vi "Close.vi"(8 "error in (no error)":errorcluster, 11 "Pound":refnum<class "Pound.lvclass">) -> (0 "error out":errorcluster)   [LabVIEW 2017, in "Pound.lvclass"]
doc: "Close reference to the pound and any watchdogs that are associated with it."
uses:
  <vilib>/NI/Software Watchdog/Pound/Pound.lvclass
  <vilib>/NI/Software Watchdog/Pound/Pound.lvclass/Pound.ctl
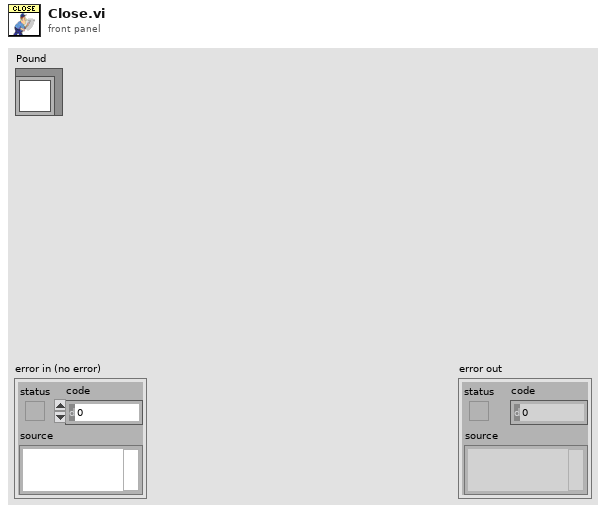
[diagram p1: front panel]
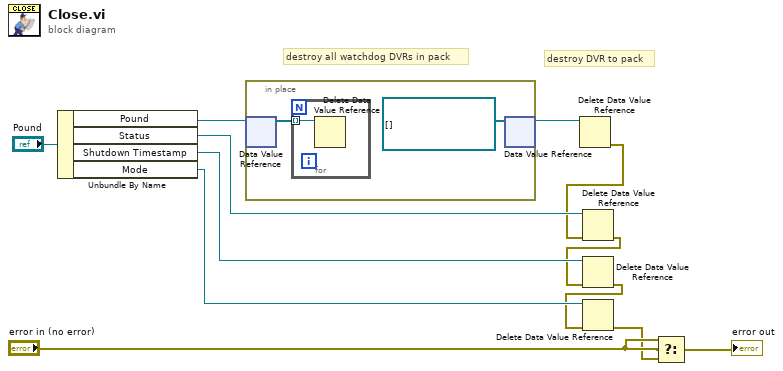
[diagram p0: block diagram]
diagram:
  # "destroy all watchdog DVRs in pack"
  # "destroy DVR to pack"
  n1 = Unbundle By Name("Pound") -> ("Pound"=w9:refnum<data-value>, "Status"=w7:refnum<data-value>, "Shutdown Timestamp"=w6:refnum<data-value>, "Mode"=w5:refnum<data-value>)
  n2 = in-place {
    n3 = in-place-dvr #1(w9) -> (w14:refnum<data-value>[])  [unwired: 1 out]
    n4 = for {
      tunnel: w14 -> [w15] mode=indexing
      n5 = Delete Data Value Reference(data value reference=w15) -> ()  [unwired: 1 in, 2 out]
    }
    n6 = in-place-dvr #1(refnum<data-value>[] [] ("data value")) -> (w8:refnum<data-value>)  [unwired: 1 out]
  }
  n7 = Delete Data Value Reference(data value reference=w8) -> (error out=w4:errorcluster)  [unwired: 1 in, 1 out]
  n8 = Delete Data Value Reference(data value reference=w7, error in=w4) -> (error out=w3:errorcluster)  [unwired: 1 out]
  n9 = Delete Data Value Reference(data value reference=w6, error in=w3) -> (error out=w2:errorcluster)  [unwired: 1 out]
  n10 = Delete Data Value Reference(data value reference=w5, error in=w2) -> (error out=w1:errorcluster)  [unwired: 1 out]
  n11 = Select(t="error in (no error)", s="error in (no error)", f=w1) -> (s? t:f=→"error out":errorcluster)
